vi "Data Server Encode Response Error.vi"(8 "error in (no error)":errorcluster, 11 "Time Stamp":timestamp) -> (0 "error out":errorcluster, 3 "Output string":string)   [LabVIEW 2011, in "Data Server VIs.lvlib"]
uses:
  Data Server VIs.lvlib
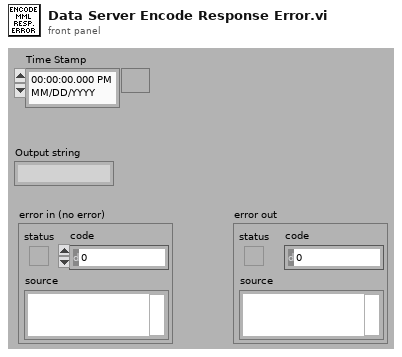
[diagram p1: front panel]
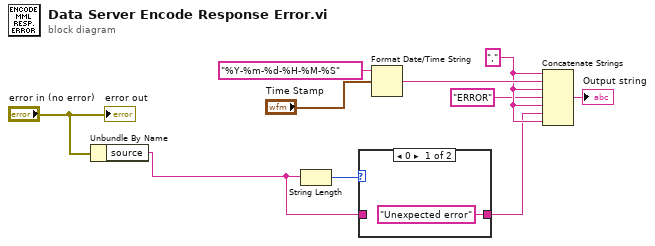
[diagram p0: block diagram]
diagram:
  w7 = "," ("string")
  n1 = Unbundle By Name("error in (no error)") -> ("source"=w1:string)
  n2 = String Length(string=w1) -> (length=w4:i32)
  n3 = case shown="0" w4 {
    tunnel: w1 -> [_ w12]
    tunnel: ["Unexpected error" ("Error description") w12] -> w3
    frame 0 {
    }
    frame 1, Default {
    }
  }
  n4 = Format Date/Time String(time format string (%c)="%Y-%m-%d-%H-%M-%S", seconds (now)="Time Stamp") -> (date/time string=w8:string)  [unwired: 1 in]
  n5 = Concatenate Strings(w7, w8, w7, "ERROR" ("string"), w7, w3, w7) -> (→"Output string":string)
  "error out" <- "error in (no error)"
